vi "Raspi_sample.vi"() -> ()   [LabVIEW 2022 SP3]
panel:
  in  "gen_button":bool
  in  "Tab Control":enum32{"Project name", "Task", "Common val"}(tab)
  in  "Project name":string="Test"
  in  "Task Names":string[](array[string])=["task_1", "task_2", "", "", "", "", "", "", "", "", "", "", "", "", "", "", "", "", "", ""]
  in  "TCP Client Task":bool
  in  "Common Valuable":string="int a;\nbool b;\npthread_t mutex;\n"
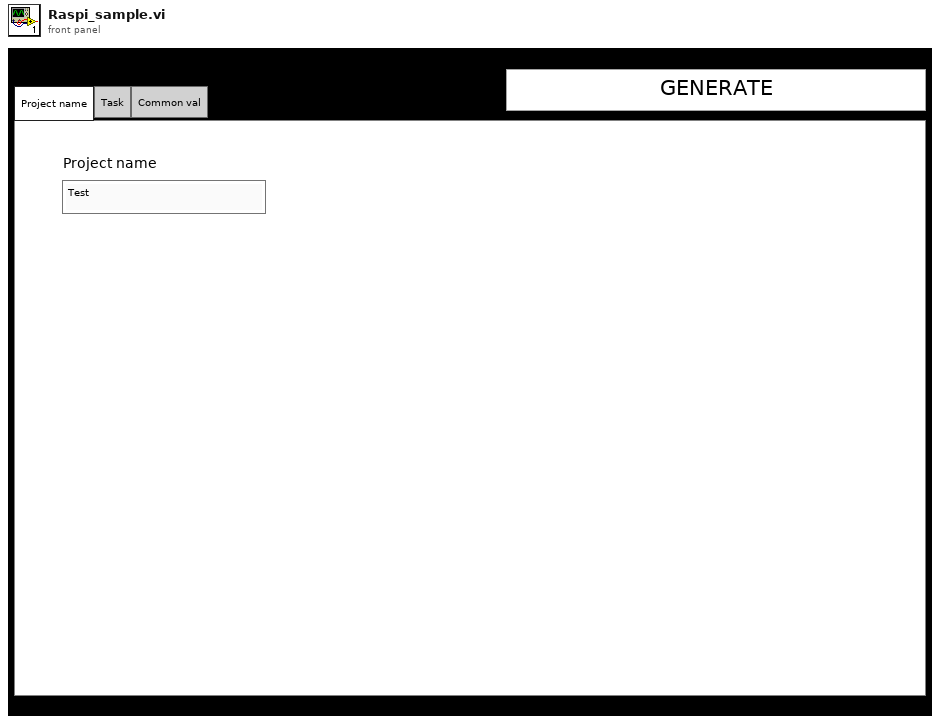
[diagram p1: front panel]
types:
  T1 = enum16{"open", "replace", "create", "open or create", "replace or create", "replace or create with confirmation"}
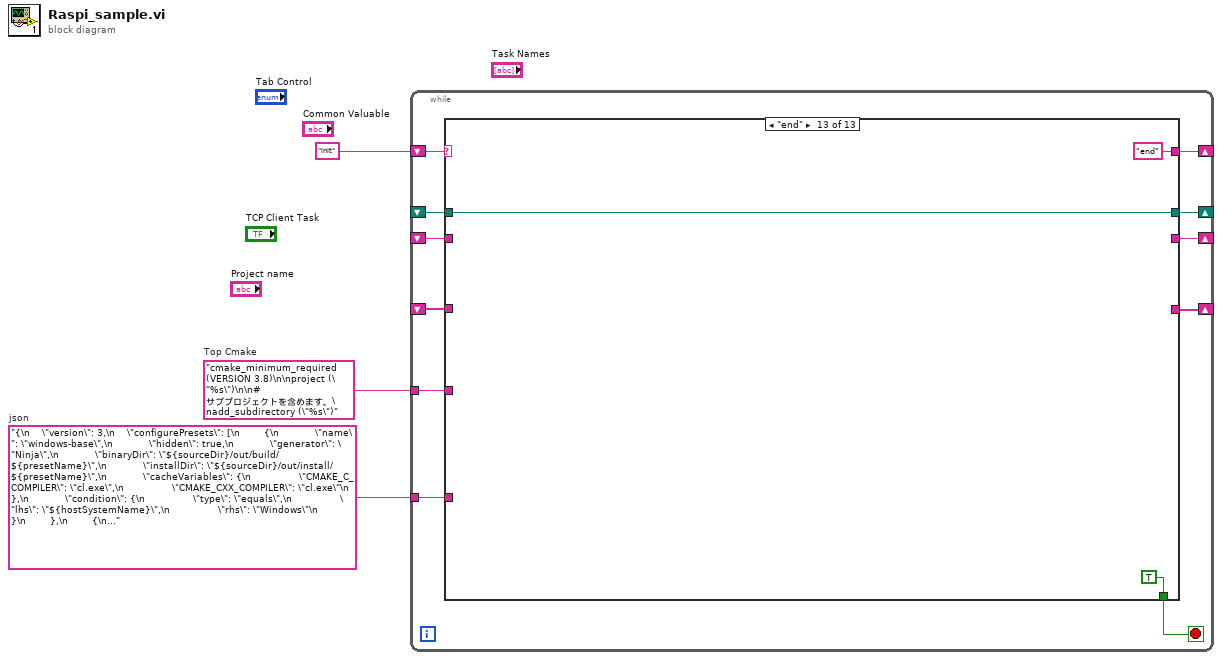
[diagram p0: block diagram]
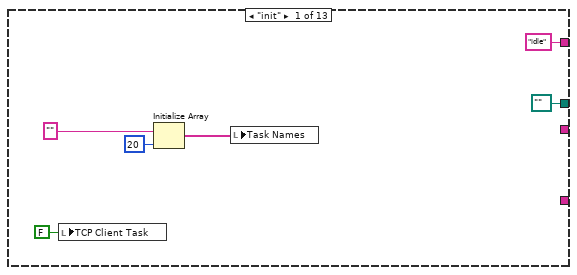
[diagram p2: hidden frame]
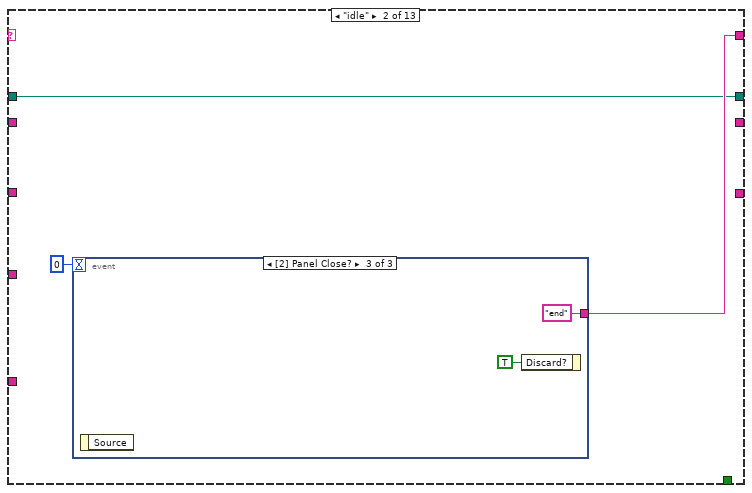
[diagram p3: hidden frame]
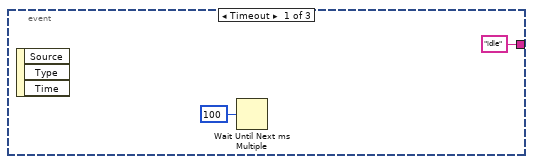
[diagram p4: hidden frame]
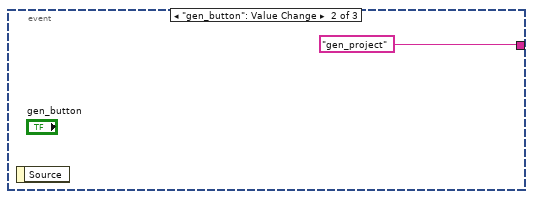
[diagram p5: hidden frame]
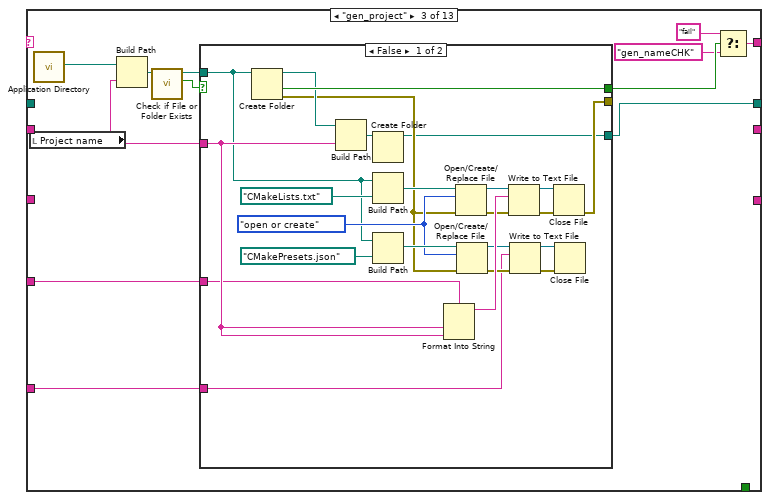
[diagram p6: hidden frame]
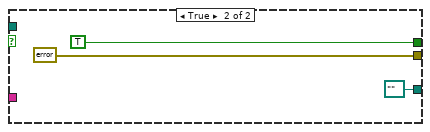
[diagram p7: hidden frame]
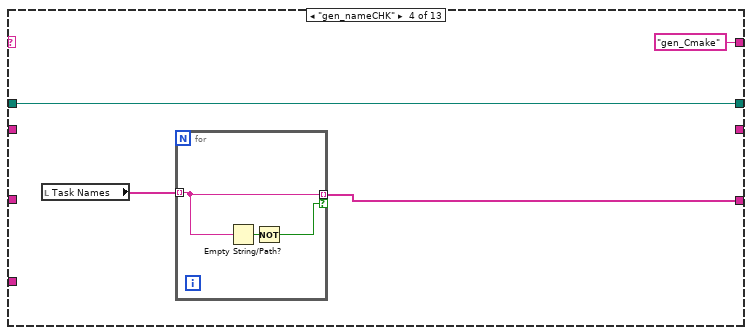
[diagram p8: hidden frame]
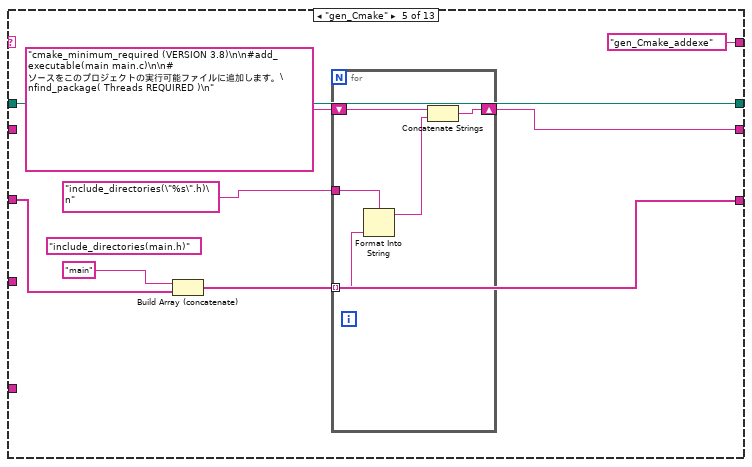
[diagram p9: hidden frame]
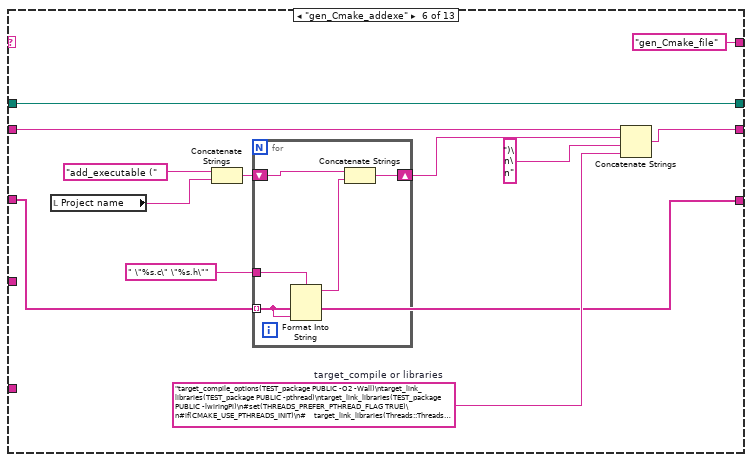
[diagram p10: hidden frame]
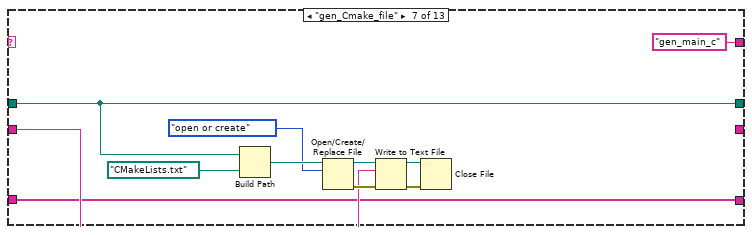
[diagram p11: hidden frame]
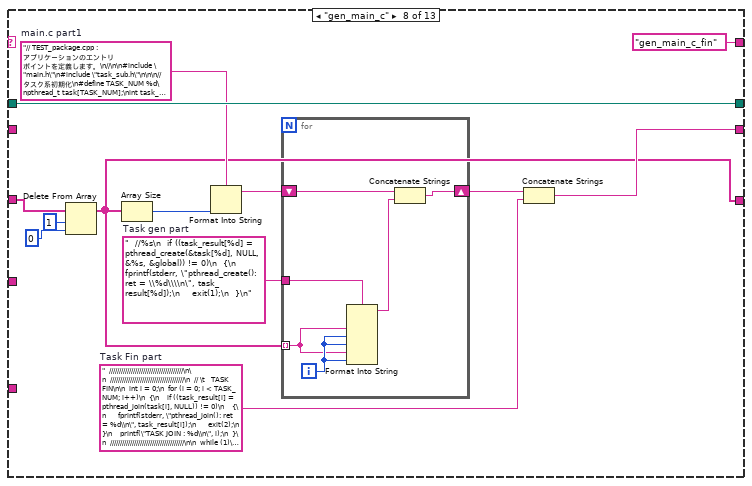
[diagram p12: hidden frame]
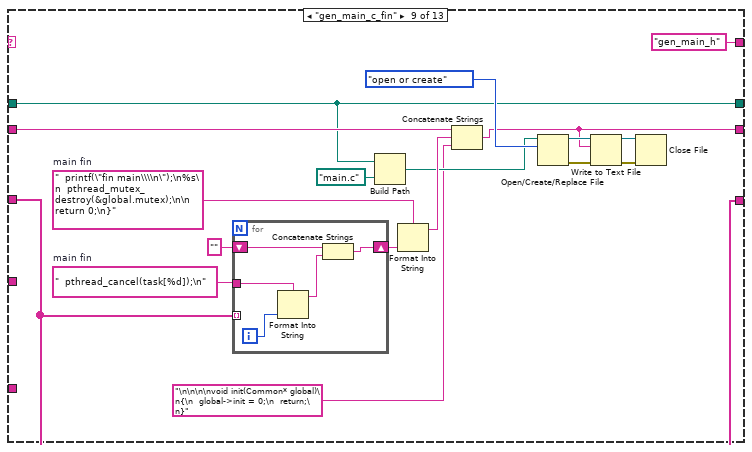
[diagram p13: hidden frame]
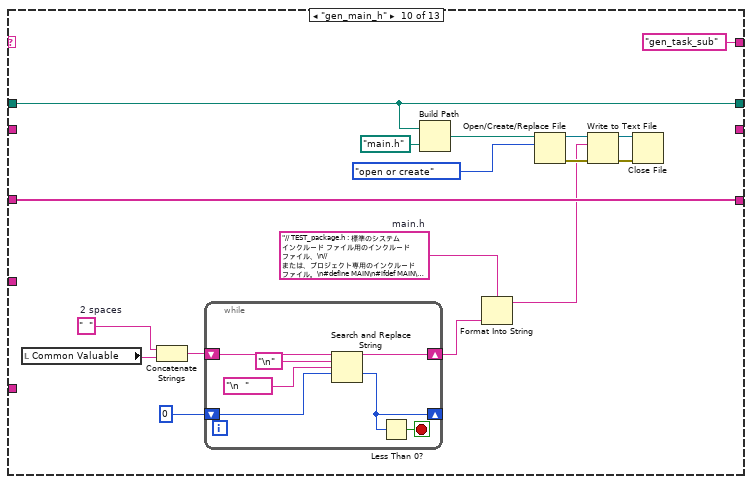
[diagram p14: hidden frame]
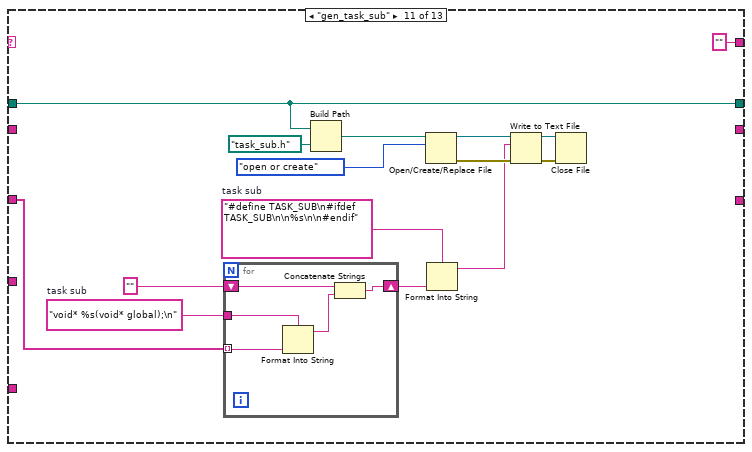
[diagram p15: hidden frame]
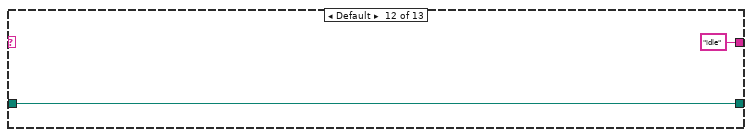
[diagram p16: hidden frame]
diagram:
  w2 = "cmake_minimum_required (VERSION 3.8)\n\nproject (\"%s\")\n\n# サブプロジェクトを含めます。\nadd_subdirectory (\"%s\")"  # Top Cmake
  w1 = "{\n    \"version\": 3,\n    \"configurePresets\": [\n        {\n            \"name\": \"windows-base\",\n            \"hidden\": true,\n            \"generator\": \"Ninja\",\n            \"binaryDir\": \"${sourceDir}/out/build/${presetName}\",\n            \"installDir\": \"${sourceDir}/out/install/${presetName}\",\n            \"cacheVariables\": {\n                \"CMAKE_C_COMPILER\": \"cl.exe\",\n                \"CMAKE_CXX_COMPILER\": \"cl.exe\"\n            },\n            \"condition\": {\n                \"type\": \"equals\",\n                \"lhs\": \"${hostSystemName}\",\n                \"rhs\": \"Windows\"\n            }\n        },\n        {\n            \"name\": \"x64-debug\",\n            \"displayName\": \"x64 Debug\",\n            \"inherits\": \"windows-base\",\n            \"architecture\": {\n                \"value\": \"x64\",\n                \"strategy\": \"external\"\n            },\n            \"cacheVariables\": {\n                \"CMAKE_BUILD_TYPE\": \"Debug\"\n            }\n        },\n        {\n            \"name\": \"x64-release\",\n            \"displayName\": \"x64 Release\",\n            \"inherits\": \"x64-debug\",\n            \"cacheVariables\": {\n                \"CMAKE_BUILD_TYPE\": \"Release\"\n            }\n        },\n        {\n            \"name\": \"x86-debug\",\n            \"displayName\": \"x86 Debug\",\n            \"inherits\": \"windows-base\",\n            \"architecture\": {\n                \"value\": \"x86\",\n                \"strategy\": \"external\"\n            },\n            \"cacheVariables\": {\n                \"CMAKE_BUILD_TYPE\": \"Debug\"\n            }\n        },\n        {\n            \"name\": \"x86-release\",\n            \"displayName\": \"x86 Release\",\n            \"inherits\": \"x86-debug\",\n            \"cacheVariables\": {\n                \"CMAKE_BUILD_TYPE\": \"Release\"\n            }\n        }\n    ]\n}\n"  # json
  n1 = while {
    shift-right: [w13] -> _
    shift-left: "init" -> [w14]
    tunnel: w2 -> [w12]
    tunnel: w1 -> [w11]
    shift-right: [w10] -> _
    shift-left: _ -> [w9]
    shift-right: [w8] -> _
    shift-left: _ -> [w7]
    shift-right: [w6] -> _
    shift-left: _ -> [w5]
    stop <- w4 stop-if-true
    n2 = case shown="\"end\"" w14 {
      tunnel: ["idle" ("f") w23 w33 "gen_Cmake" ("f") "gen_Cmake_addexe" ("f") "gen_Cmake_file" ("f") "gen_main_c" ("f") "gen_main_c_fin" ("f") "gen_main_h" ("f") "gen_task_sub" ("f") "" ("f") "idle" ("f") "end" ("f")] -> w13
      tunnel: w12 -> [_ _ w32 _ _ _ _ _ _ _ _ _ _]
      tunnel: w11 -> [_ _ w31 _ _ _ _ _ _ _ _ _ _]
      tunnel: [_ _ _ w70 w77 w89 w105 w116 w148 w174 _ _ _] -> w10
      tunnel: w9 -> [_ _ _ _ w78 w89 w105 w125 w148 w174 w195 _ _]
      tunnel: [_ _ _ _ w76 w91 _ w117 w139 _ _ _ _] -> w8
      tunnel: w7 -> [_ _ _ _ _ w94 w107 _ w150 _ _ _ _]
      tunnel: [path "" ("created path") w21 w29 w68 w75 w88 w111 w128 w138 w166 w185 w202 w206] -> w6
      tunnel: w5 -> [_ w21 _ w68 w75 w88 w111 w128 w138 w166 w185 w202 w206]
      tunnel: [_ _ _ _ _ _ _ _ _ _ _ _ TRUE] -> w4
      frame "init" {
        n3 = local write "TCP Client Task"(FALSE ("TCP Client Task")) -> ()
        n4 = Initialize Array("", 20 ("dimension size")) -> (w17:string[])
        n5 = local write "Task Names"(w17) -> ()
      }
      frame "idle" {
        n6 = event shown="[2] Panel Close?" {
          selector: _ -> [_ _ _]
          dyn-events: _ -> [_ _ _]
          timeout: 0 -> [_ _ _]
          tunnel: ["idle" "gen_project" "end"] -> w23
          event Timeout {
            n7 = event-data() -> ()  [unwired: 1 in, 3 out]
            n8 = Wait Until Next ms Multiple(millisecond multiple=u32 100) -> ()  [unwired: 1 out]
          }
          event "gen_button": Value Change {
            n9 = event-data() -> ()  [unwired: 1 in, 1 out]
          }
          event Panel Close? {
            n10 = event-data() -> ()  [unwired: 1 in, 1 out]
            n11 = event-data("Discard?"=TRUE) -> ()  [unwired: 1 in, 1 out]
          }
        }
      }
      frame "gen_project" {
        n12 = local read "Project name"() -> (w30:string)
        n13 = call <vilib>:"Application Directory.vi"() -> ("Application Directory"=w40:path)
        n14 = Build Path(base path=w40, name or relative path=w30) -> (appended path=w39:path)
        n15 = call <vilib>:"Check if File or Folder Exists.vi"("path"=w39) -> ("file or folder exists?"=w37:bool, "dup path"=w38:path)  [unwired: 8 in, 1 out]
        n16 = case shown="False" w37 {
          tunnel: w38 -> [w42 _]
          tunnel: [w64 TRUE ("cancelled")] -> w36
          tunnel: [w52 errorcluster {"status"=FALSE, "code"=0, "source"=""} ("error out")] -> _
          tunnel: w30 -> [w56 _]
          tunnel: w32 -> [w44 _]
          tunnel: w31 -> [w43 _]
          tunnel: [w41 path "" ("created path")] -> w29
          frame False {
            w48 = T1."open or create" ("operation (0:open)")
            n17 = Create Folder(path (use dialog)=w42) -> (created path=w63:path, cancelled=w64:bool, error out=w47:errorcluster)  [unwired: 2 in]
            n18 = Build Path(base path=w63, name or relative path=w56) -> (appended path=w60:path)
            n19 = Create Folder(path (use dialog)=w60) -> (created path=w41:path)  [unwired: 2 in, 2 out]
            n20 = Build Path(base path=w42, name or relative path=path "CMakeLists.txt") -> (appended path=w57:path)
            n21 = Build Path(base path=w42, name or relative path=path "CMakePresets.json") -> (appended path=w49:path)
            n22 = Format Into String(format string=w44, w56, w56) -> (resulting string=w55:string)  [unwired: 2 in, 1 out]
            n23 = Open/Create/Replace File(file path (use dialog)=w57, error in=w47, operation (0:open)=w48) -> (refnum out=w59:refnum<file>, error out=w54:errorcluster)  [unwired: 3 in, 1 out]
            n24 = Open/Create/Replace File(file path (use dialog)=w49, error in=w47, operation (0:open)=w48) -> (refnum out=w50:refnum<file>, error out=w46:errorcluster)  [unwired: 3 in, 1 out]
            n25 = Write to Text File(file (use dialog)=w59, text=w55, error in=w54) -> (refnum out=w58:refnum<file>, error out=w53:errorcluster)  [unwired: 1 in, 1 out]
            n26 = Write to Text File(file (use dialog)=w50, text=w43, error in=w46) -> (refnum out=w51:refnum<file>, error out=w45:errorcluster)  [unwired: 1 in, 1 out]
            n27 = Close File(refnum=w58, error in=w53) -> (error out=w52:errorcluster)  [unwired: 1 out]
            n28 = Close File(refnum=w51, error in=w45) -> ()  [unwired: 2 out]
          }
          frame True {
          }
        }
        n29 = Select(t="fail", s=w36, f="gen_nameCHK") -> (s? t:f=w33:string)
      }
      frame "gen_nameCHK" {
        n30 = local read "Task Names"() -> (w71:string[])
        n31 = for {
          tunnel: w71 -> [w74] mode=indexing
          tunnel: [w74] -> w70 mode=indexing if=w72
          n32 = Empty String/Path?(string/path=w74) -> (empty?=w73:bool)
          n33 = Not(x=w73) -> (.not. x?=w72:bool)
        }
      }
      frame "gen_Cmake" {
        (unwired) "include_directories(main.h)"
        n34 = Build Array (concatenate)("main", w78) -> (w77:string[])
        n35 = for {
          tunnel: w77 -> [w86] mode=indexing
          tunnel: "include_directories(\"%s\".h)\n" -> [w87]
          shift-right: [w83] -> w76
          shift-left: "cmake_minimum_required (VERSION 3.8)\n\n#add_executable(main main.c)\n\n# ソースをこのプロジェクトの実行可能ファイルに追加します。\nfind_package( Threads REQUIRED )\n" -> [w85]
          n36 = Format Into String(format string=w87, w86) -> (resulting string=w84:string)  [unwired: 2 in, 1 out]
          n37 = Concatenate Strings(w85, w84) -> (w83:string)
        }
      }
      frame "gen_Cmake_addexe" {
        w90 = "target_compile_options(TEST_package PUBLIC -O2 -Wall)\ntarget_link_libraries(TEST_package PUBLIC -pthread)\ntarget_link_libraries(TEST_package PUBLIC -lwiringPi)\n#set(THREADS_PREFER_PTHREAD_FLAG TRUE)\n#if(CMAKE_USE_PTHREADS_INIT)\n#    target_link_libraries(Threads::Threads INTERFACE -lpthread)\n#endif()\n\n\nif (CMAKE_VERSION VERSION_GREATER 3.12)\n  set_property(TARGET TEST_package PROPERTY CXX_STANDARD 20)\nendif()\n"  # target_compile or libraries
        n38 = local read "Project name"() -> (w98:string)
        n39 = Concatenate Strings("add_executable (", w98) -> (w97:string)
        n40 = for {
          shift-right: [w100] -> w93
          shift-left: w97 -> [w102]
          tunnel: " \"%s.c\" \"%s.h\"" -> [w104]
          tunnel: w89 -> [w103] mode=indexing
          n41 = Format Into String(format string=w104, w103, w103) -> (resulting string=w101:string)  [unwired: 2 in, 1 out]
          n42 = Concatenate Strings(w102, w101) -> (w100:string)
        }
        n43 = Concatenate Strings(w94, w93, ")\n\n" ("string"), w90) -> (w91:string)
      }
      frame "gen_Cmake_file" {
        n44 = Build Path(base path=w111, name or relative path=path "CMakeLists.txt") -> (appended path=w112:path)
        n45 = Open/Create/Replace File(file path (use dialog)=w112, operation (0:open)=T1."open or create") -> (refnum out=w114:refnum<file>, error out=w109:errorcluster)  [unwired: 4 in, 1 out]
        n46 = Write to Text File(file (use dialog)=w114, text=w107, error in=w109) -> (refnum out=w113:refnum<file>, error out=w108:errorcluster)  [unwired: 1 in, 1 out]
        n47 = Close File(refnum=w113, error in=w108) -> ()  [unwired: 2 out]
      }
      frame "gen_main_c" {
        w119 = "  /////////////////////////////////////\n\n  /////////////////////////////////////\n  // \t   TASK FIN\n\n  int i = 0;\n  for (i = 0; i < TASK_NUM; i++)\n  {\n    if ((task_result[i] = pthread_join(task[i], NULL)) != 0)\n    {\n      fprintf(stderr, \"pthread_join(): ret = %d\\n\", task_result[i]);\n      exit(2);\n    }\n    printf(\"TASK JOIN : %d\\n\", i);\n  }\n  /////////////////////////////////////\n\n  while (1)\n  {\n    if (global.fin >= 1)break;\n    sleep(0.5);\n  }\n"  # Task Fin part
        w122 = "  //%s\n  if ((task_result[%d] = pthread_create(&task[%d], NULL, &%s, &global)) != 0)\n  {\n    fprintf(stderr, \"pthread_create(): ret = \\%d\\\\n\", task_result[%d]);\n    exit(1);\n  }\n"  # Task gen part
        w127 = "// TEST_package.cpp : アプリケーションのエントリ ポイントを定義します。\n//\n\n#include \"main.h\"\n#include \"task_sub.h\"\n\n\n//タスク系初期化\n#define TASK_NUM %d\npthread_t task[TASK_NUM];\nint task_result[TASK_NUM];\n\n\n//メイン\nint main() {\n\n  Common global;\n  pthread_mutex_init(&global.mutex, NULL);\n  init(&global);\n\n  /////////////////////////////////////\n  // \t   TASK MAKE\n"  # main.c part1
        n48 = Delete From Array(array=w125, length=1, index=0) -> (array with subset deleted=w116:string[])  [unwired: 1 out]
        n49 = Array Size(array=w116) -> (size(s)=w126:i32)
        n50 = Format Into String(format string=w127, w126) -> (resulting string=w121:string)  [unwired: 2 in, 1 out]
        n51 = for {
          tunnel: w116 -> [w132] mode=indexing
          tunnel: w122 -> [w134]
          shift-right: [w129] -> w120
          shift-left: w121 -> [w131]
          i -> [w133]
          n52 = Format Into String(format string=w134, w132, w133, w133, w132, w133) -> (resulting string=w130:string)  [unwired: 2 in, 1 out]
          n53 = Concatenate Strings(w131, w130) -> (w129:string)
        }
        n54 = Concatenate Strings(w120, w119) -> (w117:string)
      }
      frame "gen_main_c_fin" {
        w149 = "  pthread_cancel(task[%d]);\n"  # main fin
        w146 = "  printf(\"fin main\\\\n\");\n%s\n  pthread_mutex_destroy(&global.mutex);\n\n  return 0;\n}"  # main fin
        n55 = for {
          tunnel: w149 -> [w157]
          tunnel: w148 -> [_] mode=indexing
          shift-right: [w153] -> w147
          shift-left: "" -> [w155]
          i -> [w156]
          n56 = Format Into String(format string=w157, w156) -> (resulting string=w154:string)  [unwired: 2 in, 1 out]
          n57 = Concatenate Strings(w155, w154) -> (w153:string)
        }
        n58 = Build Path(base path=w138, name or relative path=path "main.c") -> (appended path=w136:path)
        n59 = Format Into String(format string=w146, w147) -> (resulting string=w145:string)  [unwired: 2 in, 1 out]
        n60 = Concatenate Strings(w150, w145, "\n\n\n\nvoid init(Common* global)\n{\n  global->init = 0;\n  return;\n}" ("resulting string")) -> (w139:string)
        n61 = Open/Create/Replace File(file path (use dialog)=w136, operation (0:open)=T1."open or create") -> (refnum out=w144:refnum<file>, error out=w142:errorcluster)  [unwired: 4 in, 1 out]
        n62 = Write to Text File(file (use dialog)=w144, text=w139, error in=w142) -> (refnum out=w143:refnum<file>, error out=w141:errorcluster)  [unwired: 1 in, 1 out]
        n63 = Close File(refnum=w143, error in=w141) -> ()  [unwired: 2 out]
      }
      frame "gen_main_h" {
        w158 = "  "  # 2 spaces
        w164 = "// TEST_package.h : 標準のシステム インクルード ファイル用のインクルード ファイル、\n// または、プロジェクト専用のインクルード ファイル。\n#define MAIN\n#ifdef MAIN\n\n\n//#include <iostream>\n#include <stdio.h>\n#include <sys/types.h>\n#include <sys/socket.h>\n#include <netinet/in.h>\n#include <arpa/inet.h>\n#include <unistd.h>\n#include <stdlib.h>\n#include <pthread.h>\n#include <stdbool.h>\n#include <sys/select.h>\n#include <string.h>\n#include <sys/socket.h>\n#include <netdb.h>\n\n\n//タスク間で共通のグローバル\ntypedef struct \n{\n%s\n}Common;\n\nvoid init(Common* global);\n\n\n#endif //_H_MAIN\n\n// TODO: プログラムに必要な追加ヘッダーをここで参照します。\n"  # main.h
        n64 = local read "Common Valuable"() -> (w159:string)
        n65 = Concatenate Strings(w158, w159) -> (w160:string)
        n66 = while {
          shift-right: [w177] -> w162
          shift-left: w160 -> [w181]
          shift-right: [w176] -> _
          shift-left: 0 -> [w180]
          stop <- w175 stop-if-true
          n67 = Search and Replace String(input string=w181, search string="\n", replace string="\n  " ("search string"), offset=w180) -> (result string=w177:string, offset past replacement=w176:i32)  [unwired: 4 in, 2 out]
          n68 = Less Than 0?(x=w176) -> (x < 0?=w175:bool)
        }
        n69 = Build Path(base path=w166, name or relative path=path "main.h") -> (appended path=w167:path)
        n70 = Format Into String(format string=w164, w162) -> (resulting string=w161:string)  [unwired: 2 in, 1 out]
        n71 = Open/Create/Replace File(file path (use dialog)=w167, operation (0:open)=T1."open or create") -> (refnum out=w173:refnum<file>, error out=w171:errorcluster)  [unwired: 4 in, 1 out]
        n72 = Write to Text File(file (use dialog)=w173, text=w161, error in=w171) -> (refnum out=w172:refnum<file>, error out=w170:errorcluster)  [unwired: 1 in, 1 out]
        n73 = Close File(refnum=w172, error in=w170) -> ()  [unwired: 2 out]
      }
      frame "gen_task_sub" {
        w196 = "void* %s(void* global);\n"  # task sub
        w184 = "#define TASK_SUB\n#ifdef TASK_SUB\n\n%s\n\n#endif"  # task sub
        n74 = for {
          tunnel: w196 -> [w200]
          tunnel: w195 -> [w201] mode=indexing
          shift-right: [w197] -> w183
          shift-left: "" -> [w199]
          n75 = Format Into String(format string=w200, w201) -> (resulting string=w198:string)  [unwired: 2 in, 1 out]
          n76 = Concatenate Strings(w199, w198) -> (w197:string)
        }
        n77 = Build Path(base path=w185, name or relative path=path "task_sub.h") -> (appended path=w186:path)
        n78 = Open/Create/Replace File(file path (use dialog)=w186, operation (0:open)=T1."open or create") -> (refnum out=w192:refnum<file>, error out=w190:errorcluster)  [unwired: 4 in, 1 out]
        n79 = Format Into String(format string=w184, w183) -> (resulting string=w182:string)  [unwired: 2 in, 1 out]
        n80 = Write to Text File(file (use dialog)=w192, text=w182, error in=w190) -> (refnum out=w191:refnum<file>, error out=w189:errorcluster)  [unwired: 1 in, 1 out]
        n81 = Close File(refnum=w191, error in=w189) -> ()  [unwired: 2 out]
      }
      frame Default {
      }
      frame "end" {
      }
    }
  }
